vi "TCL Select Current Fragments NfragsNcriteria.vi"(3 "error in (no error)":errorcluster, 4 "criteria":T1(array[cluster]), 5 "fragments":string[](array[string])) -> (0 "error out":errorcluster, 1 "matches":string[][](array[string]), 2 "fragments out":string[](array[string]))   [LabVIEW 2010]
uses:
  TCL Global.vi
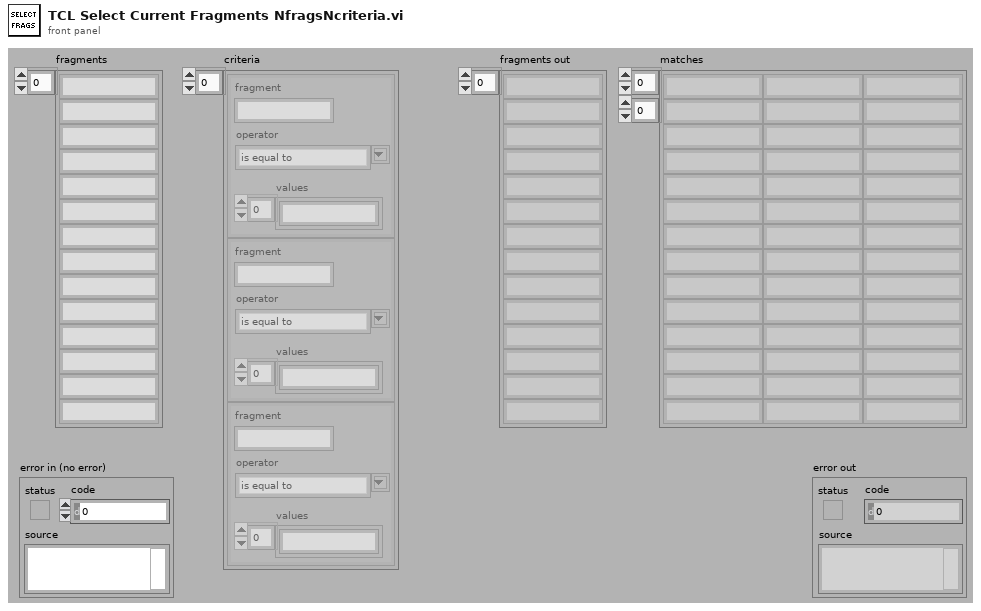
[diagram p1: front panel]
types:
  T1 = cluster{"fragment":string, "values":string[], "operator":string}[]
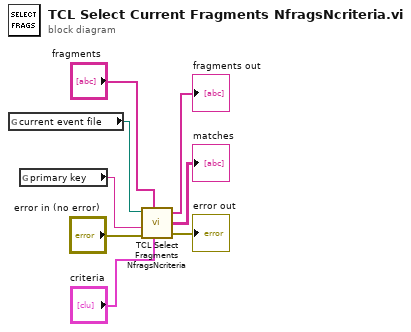
[diagram p0: block diagram]
diagram:
  n1 = global read "TCL Global.vi" "current event file"() -> (w8:path)
  n2 = global read "TCL Global.vi" "primary key"() -> (w1:string)
  n3 = call "TCL Select Fragments NfragsNcriteria.vi"("event file"=w8, "fragments"="fragments", "primary key"=w1, "criteria"="criteria", "error in (no error)"="error in (no error)") -> ("fragments out"=→"fragments out":string[], "matches"=→"matches":string[][], "error out"=→"error out":errorcluster)  [unwired: 1 in]
